vi "test2.vi"() -> ()   [LabVIEW 2017, in "ModBUS.lvlib" / "ASCII.lvclass"]
uses:
  ASCII.lvclass
panel:
  out "Data":i16[](array[numeric])
  out "Finished":bool
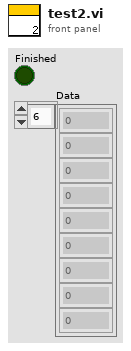
[diagram p1: front panel]
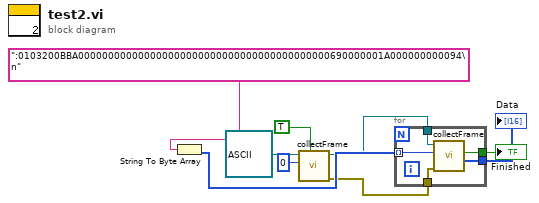
[diagram p0: block diagram]
diagram:
  n1 = String To Byte Array(string=":0103200BBA000000000000000000000000000000000000000000690000001A000000000094\n") -> (unsigned byte array=w7:u8[])
  n2 = call-dynamic "collectFrame.vi"("Reset"=TRUE, "byte"=u8 0, "ASCII in"=refnum<class "ASCII.lvclass"> refnum) -> ("error out"=w6:errorcluster, "ASCII out"=w3:refnum<class "ASCII.lvclass">)  [unwired: 4 in, 3 out]
  n3 = for {
    tunnel: w7 -> [w14] mode=indexing
    tunnel: w6 -> [w13]
    tunnel: [w12] -> w5
    tunnel: w3 -> [w11]
    tunnel: [w10] -> w1
    n4 = call-dynamic "collectFrame.vi"("error in (no error)"=w13, "byte"=w14, "ASCII in"=w11) -> ("Data"=w10:i16[], "Finished"=w12:bool)  [unwired: 4 in, 3 out]
  }
  "Finished" <- w5
  "Data" <- w1
